vi "Difference Between Angles.vi"(10 "Angle 2":dbl, 11 "Angle 1":dbl) -> (3 "Difference":dbl)   [LabVIEW 2017]
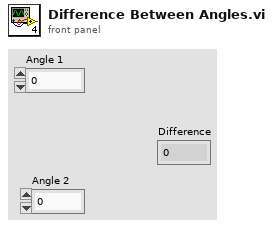
[diagram p1: front panel]
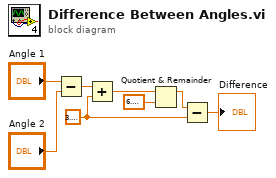
[diagram p0: block diagram]
diagram:
  w1 = 3.141592653589793
  n1 = Subtract(x="Angle 1", y="Angle 2") -> (x-y=w6:dbl)
  n2 = Add(x=w6, y=w1) -> (x+y=w5:dbl)
  n3 = Quotient & Remainder(x=w5, y=6.283185307179586) -> (x-y*floor(x/y)=w3:dbl)  [unwired: 1 out]
  n4 = Subtract(x=w3, y=w1) -> (x-y=→"Difference":dbl)
